vi "Cleanup.vi"(8 "error in (no error)":errorcluster, 11 "Node in":refnum<class "bt_Send_Notifier.lvclass">) -> (0 "error out":errorcluster, 3 "Node out":refnum<class "bt_Send_Notifier.lvclass">)   [LabVIEW 2021, in "BT.lvlib" / "bt_Send_Notifier.lvclass"]
uses:
  bt_Send_Notifier.lvclass
  bt_Send_Notifier.lvclass/bt_Send_Notifier.ctl
  With Values/Send/bt_Send_Synch_WithValues.lvclass
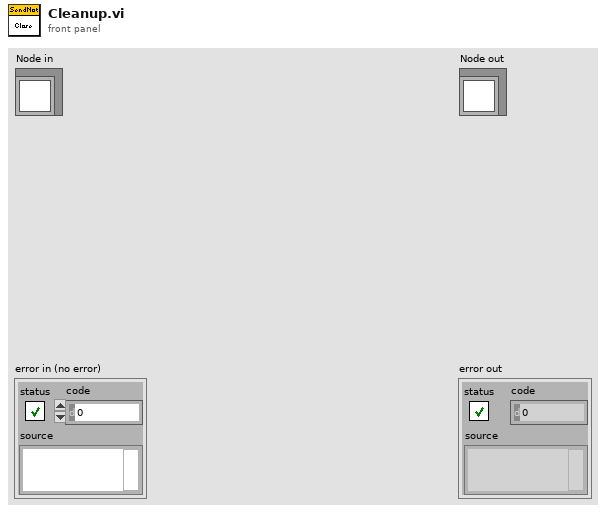
[diagram p1: front panel]
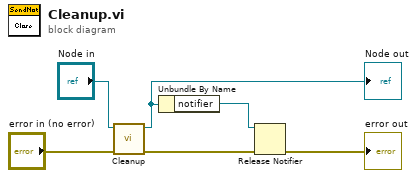
[diagram p0: block diagram]
diagram:
  n1 = call-parent "Cleanup.vi"("error in (no error)"="error in (no error)", "Node in"="Node in") -> ("error out"=w3:errorcluster, "Node out"=w4:refnum<class "bt_Send_Notifier.lvclass">)  [unwired: 8 in]
  "Node out" <- w4
  n2 = Unbundle By Name(w4) -> ("notifier"=w2:refnum<notifier>)
  n3 = Release Notifier(notifier=w2, error in (no error)=w3) -> (error out=→"error out":errorcluster)  [unwired: 1 in, 2 out]
